vi "xml single result.vi"(6 "limit type":enum16{"上限", "下限"}(ring), 7 "ABS?":bool, 8 "second result":string, 9 "single spec":dbl[](array[numeric]), 10 "TX data":string[](array[string]), 11 "RX data":string[](array[string])) -> (2 "TX array":string[](array[string]), 3 "RX array":string[](array[string]))   [LabVIEW 2011]
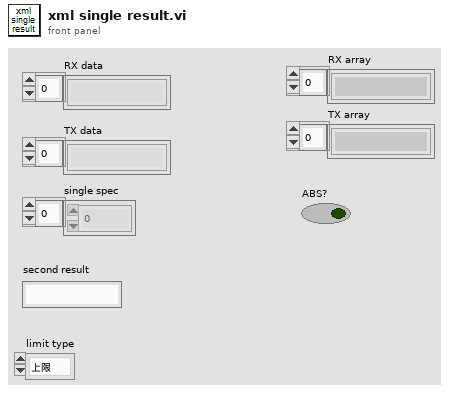
[diagram p1: front panel]
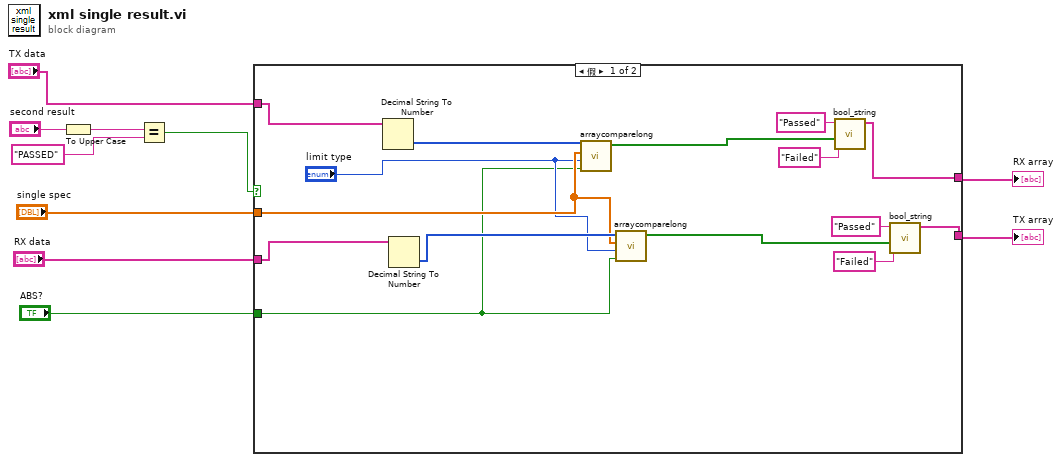
[diagram p0: block diagram]
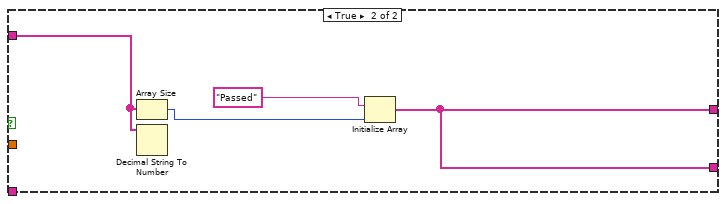
[diagram p2: hidden frame]
diagram:
  n1 = To Upper Case(1:"second result") -> (0:w9:string)
  n2 = Equal?(x=w9, y="PASSED") -> (x = y?=w7:bool)
  n3 = case shown="假" w7 {
    tunnel: "TX data" -> [w18 w27]
    tunnel: [w22 w26] -> w3
    tunnel: [w19 w26] -> w2
    tunnel: "RX data" -> [w25 _]
    tunnel: "single spec" -> [w14 _]
    tunnel: "ABS?" -> [w11 _]
    frame False {
      n4 = Decimal String To Number(string=w18) -> (number=w17:i32[])  [unwired: 2 in, 1 out]
      n5 = Decimal String To Number(string=w25) -> (number=w15:i32[])  [unwired: 2 in, 1 out]
      n6 = call "arraycomparelong.vi"("ABS?"=w11, "limit type"="limit type", "spec"=w14, "data"=w17) -> ("result"=w16:bool[])  [unwired: 7 in]
      n7 = call "arraycomparelong.vi"("ABS?"=w11, "limit type"="limit type", "spec"=w14, "data"=w15) -> ("result"=w13:bool[])  [unwired: 7 in]
      n8 = call "bool_string.vi"("boolean array"=w16, "FalseValue"="Failed", "TrueValue"="Passed") -> ("string array"=w22:string[])  [unwired: 8 in]
      n9 = call "bool_string.vi"("boolean array"=w13, "FalseValue"="Failed", "TrueValue"="Passed") -> ("string array"=w19:string[])  [unwired: 8 in]
    }
    frame True {
      n10 = Array Size(array=w27) -> (size(s)=w28:i32)
      n11 = Decimal String To Number(string=w27) -> ()  [unwired: 2 in, 2 out]
      n12 = Initialize Array("Passed" ("y"), w28) -> (w26:string[])
    }
  }
  "RX array" <- w3
  "TX array" <- w2
